vi "PI Append Group Data Fields.vi"(10 "PIM Results":T1={"Measurement Cycles"=0, "Response"="", "Measurement"={"sxFieldId"="", "sValue"="", "nDataType"=enum."Scalar", "sUnits"="", "sDisplayName"=""}, "Limit"={"Limits On"=TRUE, "Limits"=[]}, "Status Array"=[]}, 11 "Fields In":T6[](array[typedef])) -> (3 "Fields Out":T6[](array[typedef]))   [LabVIEW 2011]
uses:
  server/database/Fields/Field Record.ctl
  server/database/Fields/Field DataTypes.ctl
  server/database/Fields/Field NextItem.ctl
  TypeDefs/PI Results.ctl
  TypeDefs/PI Measurement Cluster.ctl
  TypeDefs/PI Limit Parameters.ctl
  TypeDefs/PI Limit Definition.ctl
  TypeDefs/PI Limit Comparison.ctl
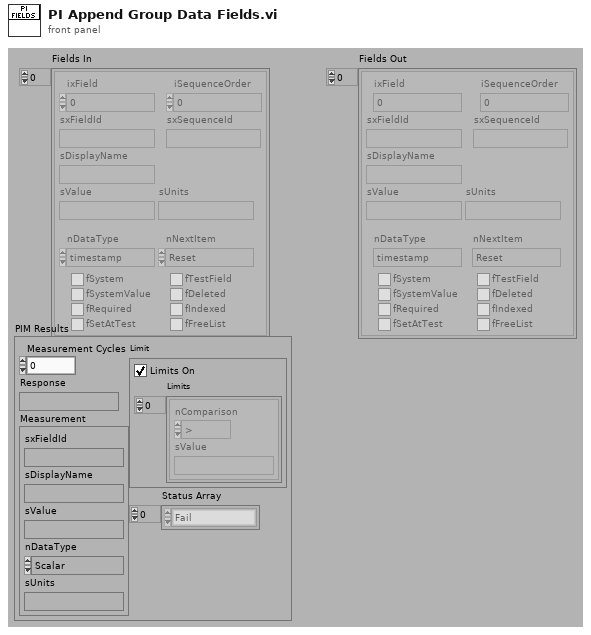
[diagram p1: front panel]
types:
  T1 = typedef "PI Results.ctl" = cluster{"Measurement Cycles":i32, "Response":string, "Measurement":T2, "Limit":T3, "Status Array":enum16{"Fail", "Pass", "Abort", "Error", "Done", "Pass by Sample", "Fail by Sample", "Pass Override", "Fail Override", "Not Tested"}[]}
  T2 = typedef "PI Measurement Cluster.ctl" = cluster{"sxFieldId":string, "sValue":string, "nDataType":enum16{"Scalar", "Enumeration"}, "sUnits":string, "sDisplayName":string}
  T3 = typedef "PI Limit Parameters.ctl" = cluster{"Limits On":bool, "Limits":T4[]}
  T4 = typedef "PI Limit Definition.ctl" = cluster{"nComparison":T5, "sValue":string}
  T5 = typedef "PI Limit Comparison.ctl" = enum16{">", ">=", "<", "<=", "<>", "="}
  T6 = typedef "Field Record.ctl" = cluster{"ixField":i32, "iSequenceOrder":i32, "sxFieldId":string, "sxSequenceId":string, "sDisplayName":string, "sValue":string, "sUnits":string, "nDataType":T7, "nNextItem":T8, "fSystem":bool, "fSystemValue":bool, "fRequired":bool, "fSetAtTest":bool, "fTestField":bool, "fDeleted":bool, "fIndexed":bool, "fFreeList":bool}
  T7 = typedef "Field DataTypes.ctl" = enum32{"text", "numeric", "list", "timestamp", "boolean"}
  T8 = typedef "Field NextItem.ctl" = enum32{"Reset", "Retain", "Auto-Increment"}
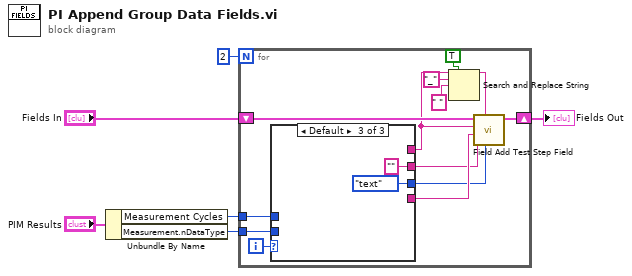
[diagram p0: block diagram]
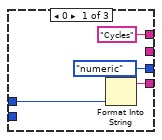
[diagram p2: hidden frame]
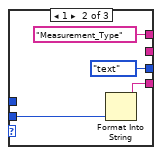
[diagram p3: hidden frame]
diagram:
  n1 = Unbundle By Name("PIM Results") -> ("Measurement Cycles"=w2:i32, "Measurement.nDataType"=w1:enum16{"Scalar", "Enumeration"})
  n2 = for {
    N: 2 -> [_]
    tunnel: w2 -> [w18]
    shift-right: [w16] -> w5
    shift-left: "Fields In" -> [w17]
    tunnel: w1 -> [w12]
    i -> [w19]
    n3 = case shown="Default" w19 {
      tunnel: w18 -> [w20 _ _]
      tunnel: ["Cycles" ("Field_ID") "Measurement_Type" ("Field_ID") _] -> w7
      tunnel: [Field_DataTypes."numeric" ("Data Type") Field_DataTypes."text" ("Data Type") Field_DataTypes."text" ("Data Type")] -> w14
      tunnel: [w22 w24 _] -> w15
      tunnel: [_ _ "" ("Field_ID")] -> w13
      tunnel: w12 -> [_ w25 _]
      frame 0 {
        n4 = Format Into String(w20) -> (resulting string=w22:string)  [unwired: 3 in, 1 out]
      }
      frame 1 {
        n5 = Format Into String(w25) -> (resulting string=w24:string)  [unwired: 3 in, 1 out]
      }
      frame Default {
      }
    }
    n6 = Search and Replace String(replace all?=TRUE ("replace all? (F)"), input string=w7, search string="_", replace string=" " ("replace string (\"\")")) -> (result string=w8:string)  [unwired: 1 in, 6 out]
    n7 = call "Field Add Test Step Field.vi"("nDataType"=w14, "sDisplayName"=w8, "sUnits"=w13, "sValue"=w15, "sxFieldId"=w7, "Fields In"=w17) -> ("Fields Out"=w16:T6[])  [unwired: 5 out]
  }
  "Fields Out" <- w5
